vi "Configure Slew Rate (All).vi"(0 "VISA resource name":refnum<visa-resource-name>, 5 "Voltage Slew Rate (0 V per sec)":dbl format="%#.6f", 7 "Current Slew Rate (0 A per sec)":dbl format="%#.6f", 9 "Power Slew Rate (0 W per sec)":dbl format="%#.6f", 11 "error in (no error)":errorcluster, 12 "Resistance Slew Rate (0 Ohms per sec)":dbl format="%#.6f") -> (4 "VISA resource name out":refnum<visa-resource-name>, 15 "error out":errorcluster)   [LabVIEW 2012, in "NH Research Regenerative Test Series.lvlib"]
doc: "Sets the slew rate for all programmed changes in the output of the module. This command programs both positive and negative going slew rates. Although any slew rate value may be entered, the module selects a slew rate that is closest to the programmed value."
uses:
  <instrlib>/NH Research Regenerative Test Series/NH Research Regenerative Test Series.lvlib
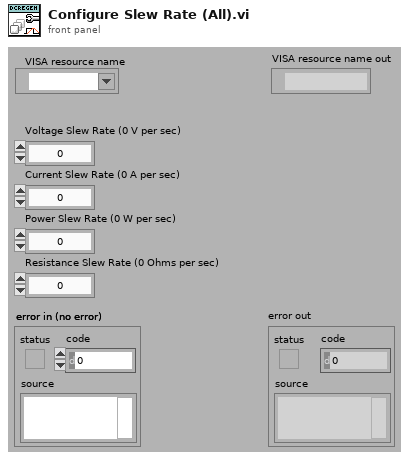
[diagram p1: front panel]
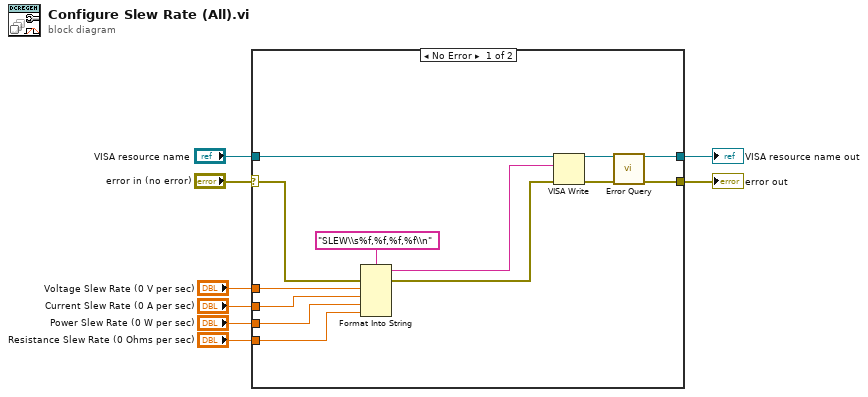
[diagram p0: block diagram]
diagram:
  n1 = case shown="No Error" "error in (no error)" {
    selector: "error in (no error)" -> [w15 w23]
    tunnel: "VISA resource name" -> [w21 w22]
    tunnel: [w20 w22] -> w7
    tunnel: [w19 w23] -> w6
    tunnel: "Voltage Slew Rate (0 V per sec)" -> [w16 _]
    tunnel: "Current Slew Rate (0 A per sec)" -> [w11 _]
    tunnel: "Power Slew Rate (0 W per sec)" -> [w10 _]
    tunnel: "Resistance Slew Rate (0 Ohms per sec)" -> [w9 _]
    frame No Error {
      n2 = Format Into String(format string="SLEW\\s%f,%f,%f,%f\\n", error in=w15, w16, w11, w10, w9) -> (resulting string=w13:string, error out=w14:errorcluster)  [unwired: 1 in]
      n3 = VISA Write(VISA resource name=w21, write buffer=w13, error in (no error)=w14) -> (VISA resource name out=w18:refnum<visa-resource-name>, error out=w17:errorcluster)  [unwired: 1 out]
      n4 = call <instrlib>:"Error Query.vi"("VISA resource name"=w18, "error in (no error)"=w17) -> ("VISA resource name out"=w20:refnum<visa-resource-name>, "error out"=w19:errorcluster)  [unwired: 10 in, 2 out]
    }
    frame Error {
    }
  }
  "error out" <- w6
  "VISA resource name out" <- w7
